vi "svc_Convert Array of Peaks to X and Y Arrays.vi"(4 "peaks":cluster{"frequency [Hz]":dbl, "amplitude":dbl}[](array[cluster])) -> (1 "Y":dbl[](array[numeric]), 2 "X":dbl[](array[numeric]))   [LabVIEW 2017]
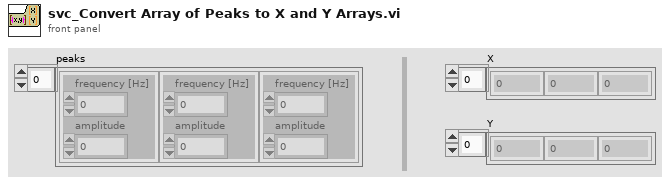
[diagram p1: front panel]
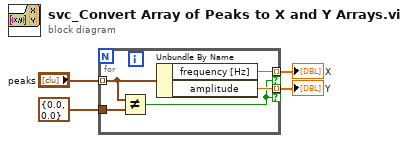
[diagram p0: block diagram]
diagram:
  n1 = for {
    tunnel: "peaks" -> [w8] mode=indexing
    tunnel: cluster{"frequency [Hz]":dbl, "amplitude":dbl} {"frequency [Hz]"=0.0, "amplitude"=0.0} -> [w9]
    tunnel: [w7] -> w3 mode=indexing if=w5
    tunnel: [w6] -> w4 mode=indexing if=w5
    n2 = Not Equal?(x=w8, y=w9) -> (x != y?=w5:bool)
    n3 = Unbundle By Name(w8) -> ("frequency [Hz]"=w7:dbl, "amplitude"=w6:dbl)
  }
  "Y" <- w4
  "X" <- w3
